vi "Get Class Information.vi"(7 "Object":refnum<class>, 8 "error in (no error)":errorcluster, 11 "CConfig Variant Accessor in":refnum<class "CConfig Variant Accessor.lvclass">) -> (0 "error out":errorcluster, 2 "Class default data":variant[](array[variant]), 3 "CConfig Variant Accessor out":refnum<class "CConfig Variant Accessor.lvclass">, 4 "Class versions":T1(array[cluster]), 5 "Object (dup)":refnum<class>, 6 "Class name":string)   [LabVIEW 2013, in "CConfig Variant Accessor.lvclass"]
doc: "Copyright 2018, Carya Automatisering, Wiebe Walstra."
uses:
  CConfig Variant Accessor.lvclass
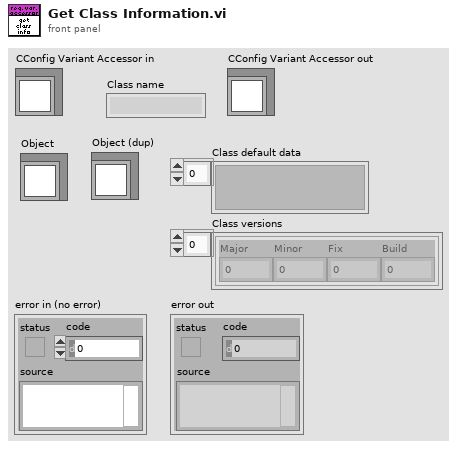
[diagram p1: front panel]
types:
  T1 = cluster{"Major":u16, "Minor":u16, "Fix":u16, "Build":u16}[]
  T2 = cluster{"Major":u16, "Minor":u16, "Fix":u16, "Build":u16}
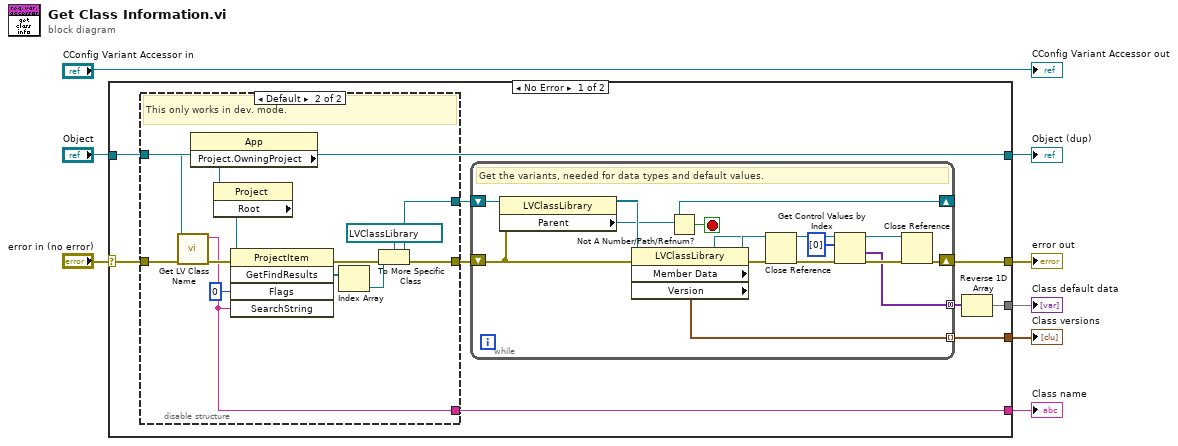
[diagram p0: block diagram]
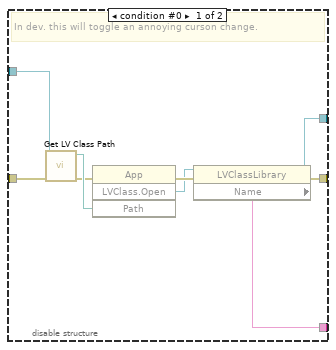
[diagram p2: hidden frame]
diagram:
  n1 = case shown="No Error" "error in (no error)" {
    selector: "error in (no error)" -> [w15 w54]
    tunnel: [w12 w54] -> w7
    tunnel: "Object" -> [w14 w53]
    tunnel: [w9 _] -> w5
    tunnel: [w16 _] -> w4
    tunnel: [w13 _] -> w3
    tunnel: [w14 w53] -> w1
    frame No Error {
      n2 = disable-structure shown="Default" {
        disable-tunnel: w15 -> [w38 w52]
        disable-tunnel: w14 -> [w37 w51]
        disable-tunnel: [w34 w47] -> w13
        disable-tunnel: [w32 w41] -> w12
        disable-tunnel: [w31 w40] -> w11
        frame condition #0 {
          # "In dev. this will toggle an annoying curson change."
          n3 = call <vilib>:"Get LV Class Path.vi"("error in (no error)"=w38, "object"=w37) -> ("error out"=w33:errorcluster, "class path"=w39:path)  [unwired: 8 in]
          n4 = invoke class="App" method="LVClass.Open"(error in=w33, "Path"=w39) -> (error out=w36:errorcluster, "LVClass.Open"=w35:refnum<vi>)  [unwired: 2 in, 2 out]
          n5 = property class="LVClassLibrary"(reference=w35, error in=w36) -> (reference out=w31:refnum<vi>, error out=w32:errorcluster, "Name"=w34:string)
        }
        frame condition #1 (active) {
          # "This only works in dev. mode."
          n6 = call <vilib>:"Get LV Class Name.vi"("error in (no error)"=w52, "object"=w51) -> ("error out"=w50:errorcluster, "class name"=w47:string)  [unwired: 8 in]
          n7 = property class="App"() -> ("Project.OwningProject"=w49:refnum<vi>)  [unwired: 2 in, 2 out]
          n8 = property class="Project"(reference=w49) -> ("Root"=w48:refnum<vi>)  [unwired: 1 in, 2 out]
          n9 = invoke class="ProjectItem" method="GetFindResults"(reference=w48, error in=w50, "Flags"=0, "SearchString"=w47) -> (error out=w45:errorcluster, "GetFindResults"=w46:refnum<vi>[])  [unwired: 1 in, 3 out]
          n10 = Index Array(array=w46) -> (element=w44:refnum<vi>)  [unwired: 1 in]
          n11 = To More Specific Class(target class=refnum<vi> refnum ("Parent"), reference=w44, error in=w45) -> (specific class reference=w40:refnum<vi>, error out=w41:errorcluster)
        }
      }
      n12 = while {
        tunnel: [w30] -> w9 mode=indexing
        shift-right: [w21] -> _
        shift-left: w11 -> [w26]
        shift-right: [w18] -> _
        shift-left: w12 -> [w22]
        tunnel: [w24] -> w10 mode=concatenating
        stop <- w20 stop-if-true
        # "Get the variants, needed for data types and default values."
        n13 = property class="LVClassLibrary"(reference=w26, error in=w22) -> (reference out=w23:refnum<vi>, "Parent"=w21:refnum<vi>)  [unwired: 1 out]
        n14 = property class="LVClassLibrary"(reference=w23, error in=w22) -> (reference out=w28:refnum<vi>, error out=w29:errorcluster, "Member Data"=w17:refnum<vi>, "Version"=w30:T2)
        n15 = Not A Number/Path/Refnum?(number/path/refnum=w21) -> (NaN/Path/Refnum?=w20:bool)
        n16 = Close Reference(reference=w28, error in (no error)=w29) -> (error out=w25:errorcluster)
        n17 = Get Control Values by Index(0:w17, 1:i32[] [0] ("control indexes"), 3:w25) -> (10:w24:variant[], 11:w19:errorcluster)
        n18 = Close Reference(reference=w17, error in (no error)=w19) -> (error out=w18:errorcluster)
      }
      n19 = Reverse 1D Array(array=w10) -> (reversed array=w16:variant[])
    }
    frame Error {
    }
  }
  "error out" <- w7
  "Class versions" <- w5
  "Class default data" <- w4
  "Class name" <- w3
  "Object (dup)" <- w1
  "CConfig Variant Accessor out" <- "CConfig Variant Accessor in"
